vi "Robot Global Data.vi"() -> ()   [LabVIEW 2016]
doc: "This global VI can contain as many global variables as you need. Place a control on the panel, give it a good name. To read or write to it from a VI, drag the icon to the diagram of that VI. You can also drag from the project. Click on the node to change which global you access. You shouldn't have multiple locations writing to a global or it will cause a race-condition."
uses:
  <vilib>/Rock Robotics/WPI/Camera/WPI_CameraImageSize.ctl
  <vilib>/Rock Robotics/WPI/DriverStation/WPI_DriverStationRobotMode2.ctl
  dash_to_rio_cluster.ctl
  Auto modes.ctl
  Shifter override.ctl
  rio_to_dash_cluster.ctl
panel:
  out "Pixy":T1
  out "Lift power":dbl
  out "Lift button":bool
  in  "Lift Current":dbl
  in  "Lift Switch?":bool
  out "Robot to DS":T2
  out "DS to robot":T3
  in  "Shooter active?":bool
  in  "Drive":T6
  in  "Shooter speed":dbl
  in  "Robot Mode":T7
  in  "image size":T8=enum."320x240"
  in  "Enable Vision":bool
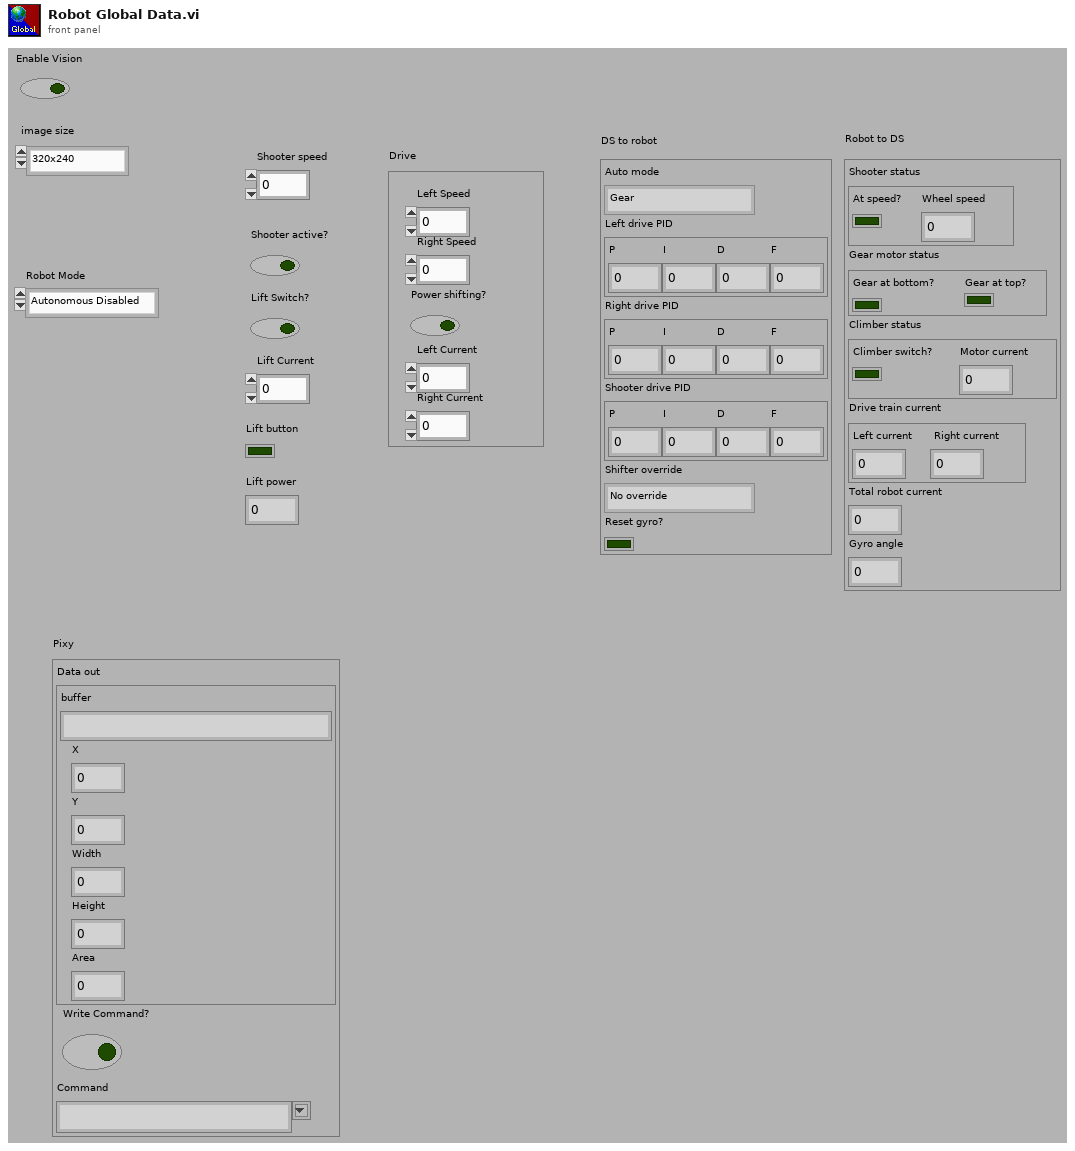
[diagram p1: front panel]
types:
  T1 = cluster{"Data out":cluster{"buffer":string, "X":i32, "Y":i32, "Width":i32, "Height":i32, "Area":dbl}, "Write Command?":bool, "Command":string}
  T2 = typedef "rio_to_dash_cluster.ctl" = cluster{"Shooter status":cluster{"At speed?":bool, "Wheel speed":dbl}, "Gear motor status":cluster{"Gear at bottom?":bool, "Gear at top?":bool}, "Climber status":cluster{"Climber switch?":bool, "Motor current":dbl}, "Drive train current":cluster{"Left current":dbl, " Right current":dbl}, "Total robot current":dbl, "Gyro angle":dbl}
  T3 = typedef "dash_to_rio_cluster.ctl" = cluster{"Auto mode":T4, "Left drive PID ":cluster{"P":dbl, "I":dbl, "D":dbl, "F":dbl}, "Right drive PID ":cluster{"P":dbl, "I":dbl, "D":dbl, "F":dbl}, "Shooter drive PID ":cluster{"P":dbl, "I":dbl, "D":dbl, "F":dbl}, "Shifter override":T5, "Reset gyro?":bool}
  T4 = typedef "Auto modes.ctl" = enum16{"Gear", "Shooter", "Gear + Shooter", "None", "Shooter + Cheesecake", "Shooter + Bin"}
  T5 = typedef "Shifter override.ctl" = enum16{"No override", "High ", "Low"}
  T6 = cluster{"Left Speed":dbl, "Right Speed":dbl, "Power shifting?":bool, "Left Current":dbl, "Right Current":dbl}
  T7 = typedef "WPI_DriverStationRobotMode2.ctl" = enum16{"Autonomous Disabled", "Autonomous Enabled", "Teleop Disabled", "Teleop Enabled", "Disconnected", "Finish", "Test Disabled", "Test Enabled", "Emergency Stopped"}
  T8 = typedef "WPI_CameraImageSize.ctl" = enum16{"640x480", "320x240", "160x120", "Custom"}
diagram:
